vi "Is Sleeping.vi"(8 "error in (no error)":errorcluster, 11 "ISleepableCellPhone in":refnum<class "ISleepableCellPhone.lvclass">) -> (0 "error out":errorcluster, 2 "IsSleeping":bool, 3 "ISleepableCellPhone out":refnum<class "ISleepableCellPhone.lvclass">)   [LabVIEW 2009, in "ISleepableCellPhone.lvclass"]
uses:
  ISleepableCellPhone.lvclass
  CellPhone.lvclass
  Source/IUnknown Class/IUnknown.lvclass
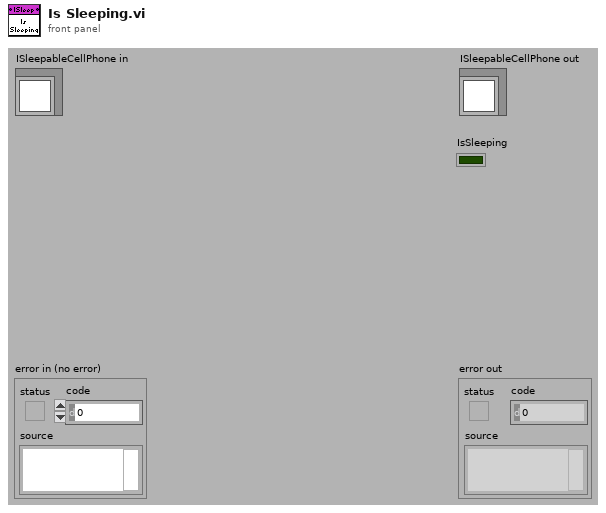
[diagram p1: front panel]
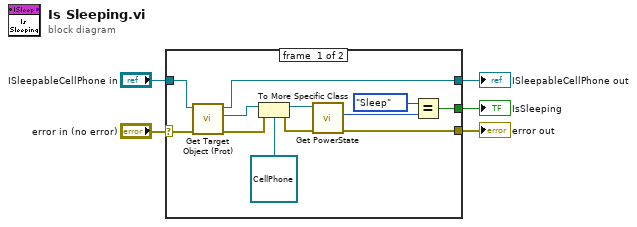
[diagram p0: block diagram]
diagram:
  n1 = case shown="No Error" "error in (no error)" {
    selector: "error in (no error)" -> [w6 w18]
    tunnel: "ISleepableCellPhone in" -> [w17 w19]
    tunnel: [w16 w19] -> w4
    tunnel: [w12 w18] -> w3
    tunnel: [w7 _] -> w2
    frame #0 {
      n2 = call "Get Target Object (Prot).vi"("error in (no error)"=w6, "IUnknown in"=w17) -> ("error out"=w10:errorcluster, "Target Object"=w11:refnum<class "Interfaceable.lvclass">, "IUnknown out"=w16:refnum<class "ISleepableCellPhone.lvclass">)  [unwired: 7 in]
      n3 = To More Specific Class(target class=refnum<class "CellPhone.lvclass"> refnum ("CellPhone"), reference=w11, error in=w10) -> (specific class reference=w14:refnum<class "CellPhone.lvclass">, error out=w13:errorcluster)
      n4 = call "Get PowerState.vi"("error in (no error)"=w13, "CellPhone in"=w14) -> ("error out"=w12:errorcluster, "PowerState"=w8:enum16{"Off", "Sleep", "On"})  [unwired: 7 in, 1 out]
      n5 = Equal?(x=enum16{"Off", "Sleep", "On"}."Sleep" ("PowerState"), y=w8) -> (x = y?=w7:bool)
    }
    frame #1 {
    }
  }
  "error out" <- w3
  "ISleepableCellPhone out" <- w4
  "IsSleeping" <- w2
